vi "Configure Measurement Snapshot.vi"(8 "error in (no error)":errorcluster, 9 "Snapshot Action (0: Take Snapshot)":i32(ring) items=["Take Snapshot", "Clear Snapshot"], 10 "Snapshot Source (0: Channel 1)":i32(ring) items=["Channel 1"=0, "Channel 2"=1, "Math"=4], 11 "VISA resource name":refnum<visa-resource-name>) -> (0 "error out":errorcluster, 3 "VISA resource name out":refnum<visa-resource-name>)   [LabVIEW 2012, in "Tektronix TDS 200 1000 2000 Series.lvlib"]
doc: "Configures the snapshot source and run snapshot.\n\n<b>Note(s):</b>\nThis VI is only applicable for TBS1000B and TBS1000B-EDU series models."
uses:
  <instrlib>/Tektronix TDS 200 1000 2000 Series/Tektronix TDS 200 1000 2000 Series.lvlib
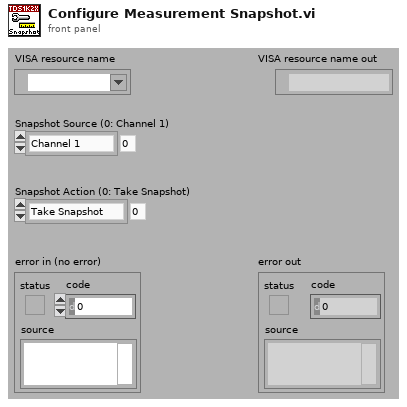
[diagram p1: front panel]
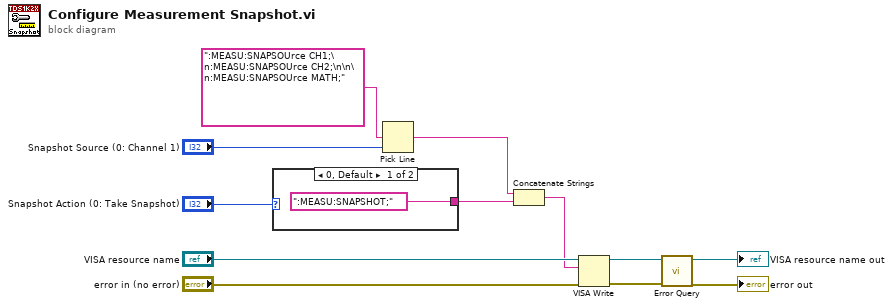
[diagram p0: block diagram]
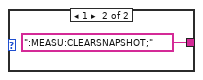
[diagram p2: hidden frame]
diagram:
  n1 = case shown="0, Default" "Snapshot Action (0: Take Snapshot)" {
    tunnel: [":MEASU:SNAPSHOT;" ":MEASU:CLEARSNAPSHOT;"] -> w3
    frame 0, Default {
    }
    frame 1 {
    }
  }
  n2 = Pick Line(multi-line string=":MEASU:SNAPSOUrce CH1;\n:MEASU:SNAPSOUrce CH2;\n\n\n:MEASU:SNAPSOUrce MATH;", line index="Snapshot Source (0: Channel 1)") -> (output string=w2:string)  [unwired: 1 out]
  n3 = Concatenate Strings(w2, w3) -> (w1:string)
  n4 = VISA Write(VISA resource name="VISA resource name", write buffer=w1, error in (no error)="error in (no error)") -> (VISA resource name out=w5:refnum<visa-resource-name>, error out=w4:errorcluster)  [unwired: 1 out]
  n5 = call <instrlib>:"Error Query.vi"("error in (no error)"=w4, "VISA resource name"=w5) -> ("error out"=→"error out":errorcluster, "VISA resource name out"=→"VISA resource name out":refnum<visa-resource-name>)  [unwired: 8 out]
